vi "Step jsObject Array.vi"(8 "error in (no error)":errorcluster, 9 "STEPS (none)":T1[](array[typedef]), 10 "Steps jsObject Array Name (\"STEPS\")":string="STEPS", 11 "Previous String (\"\")":string) -> (0 "error out":errorcluster, 2 "Steps jsObject Array":string, 3 "Step Definition":string)   [LabVIEW 2011]
uses:
  Step Record.ctl
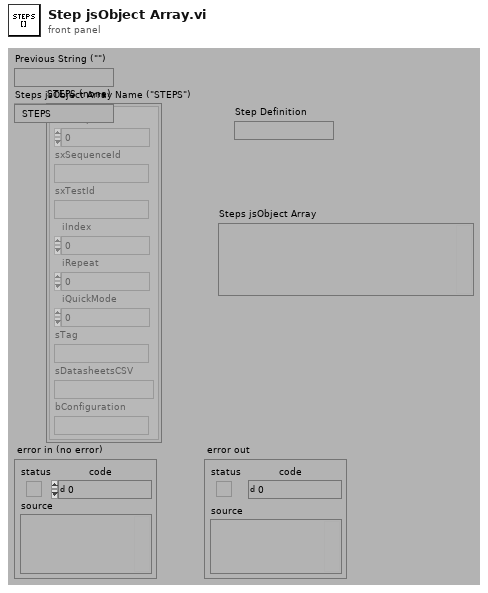
[diagram p1: front panel]
types:
  T1 = typedef "Step Record.ctl" = cluster{"ixStep":i32, "sxSequenceId":string, "sxTestId":string, "iIndex":i32, "iRepeat":i32, "iQuickMode":i32, "sTag":string, "sDatasheetsCSV":string, "bConfiguration":string}
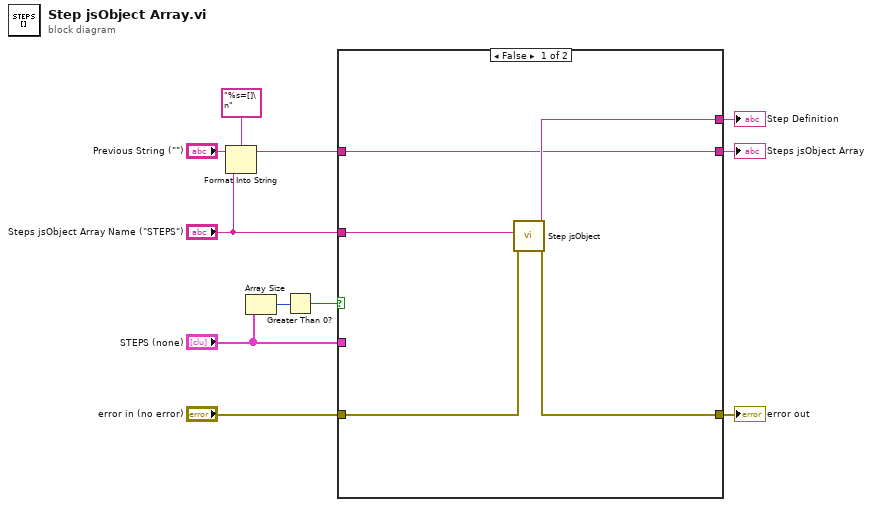
[diagram p0: block diagram]
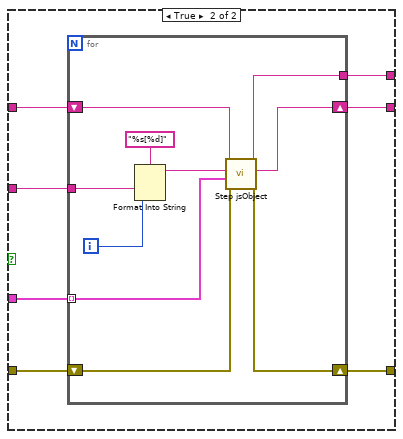
[diagram p2: hidden frame]
diagram:
  n1 = Format Into String(format string="%s=[]\n", initial string="Previous String (\"\")", "Steps jsObject Array Name (\"STEPS\")") -> (resulting string=w10:string)  [unwired: 1 in, 1 out]
  n2 = Array Size(array="STEPS (none)") -> (size(s)=w9:i32)
  n3 = Greater Than 0?(x=w9) -> (x > 0?=w8:bool)
  n4 = case shown="False" w8 {
    tunnel: w10 -> [w12 w23]
    tunnel: "error in (no error)" -> [w16 w22]
    tunnel: [w12 w21] -> w4
    tunnel: [w15 w20] -> w3
    tunnel: "Steps jsObject Array Name (\"STEPS\")" -> [w13 w19]
    tunnel: [w14 w18] -> w5
    tunnel: "STEPS (none)" -> [_ w17]
    frame False {
      n5 = call "Step jsObject.vi"("error in (no error)"=w16, "Step jsObject Name (\"\")"=w13) -> ("error out"=w15:errorcluster, "STEP definition"=w14:string)  [unwired: 2 in, 6 out]
    }
    frame True {
      n6 = for {
        tunnel: w17 -> [w26] mode=indexing
        shift-right: [w24] -> w21
        shift-left: w23 -> [w33]
        shift-right: [w31] -> w20
        shift-left: w22 -> [w32]
        tunnel: w19 -> [w28]
        tunnel: [w25] -> w18
        i -> [w27]
        n7 = Format Into String(format string="%s[%d]", w28, w27) -> (resulting string=w29:string)  [unwired: 2 in, 1 out]
        n8 = call "Step jsObject.vi"("error in (no error)"=w32, "Step Record (empty)"=w26, "Step jsObject Name (\"\")"=w29, "Previous String (\"\")"=w33) -> ("error out"=w31:errorcluster, "Step jsObject"=w24:string, "STEP definition"=w25:string)  [unwired: 5 out]
      }
    }
  }
  "Steps jsObject Array" <- w4
  "error out" <- w3
  "Step Definition" <- w5
